vi "WaitAdjust.vi"(9 "PassthroughTime_SEC":dbl=-1.0, 10 "MaxAdjustment_MS":dbl=5.0, 11 "DesiredLoopTime_MS":dbl=20.0) -> (2 "AdjustedWaitTime_MS":u32, 3 "Offset_MS":dbl)   [LabVIEW 2019, in "Trajectory_Library.lvlib"]
doc: "This routine fine tunes the wait time for a loop to attempt to provide the loop with more consistent timing and lower jitter. \n\nInputs:\n -- Desired Loop time -- Int32 -- Desired loop time in milliseconds. (Optional. Default: 20.0)\n -- MaxAdjustment -- Int32 -- Maximum time in milliseconds to adjust the wait time. (Optional. Default: 5.0)\n -- PassthroughTime -- double float -- Elapsed time clock. (Optional. Default: Read FPGA clock)\n\nOutputs:\n -- Adjusted Wait Time -- Uint32 -- Updated wait time in milliseconds to feed to the wait VI.\n - Offset MS -- double float -- Current value of accumulated loop time error."
uses:
  Trajectory_Library.lvlib
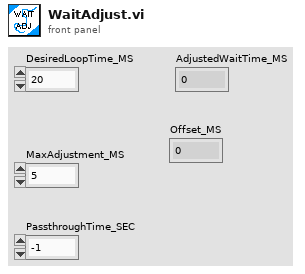
[diagram p1: front panel]
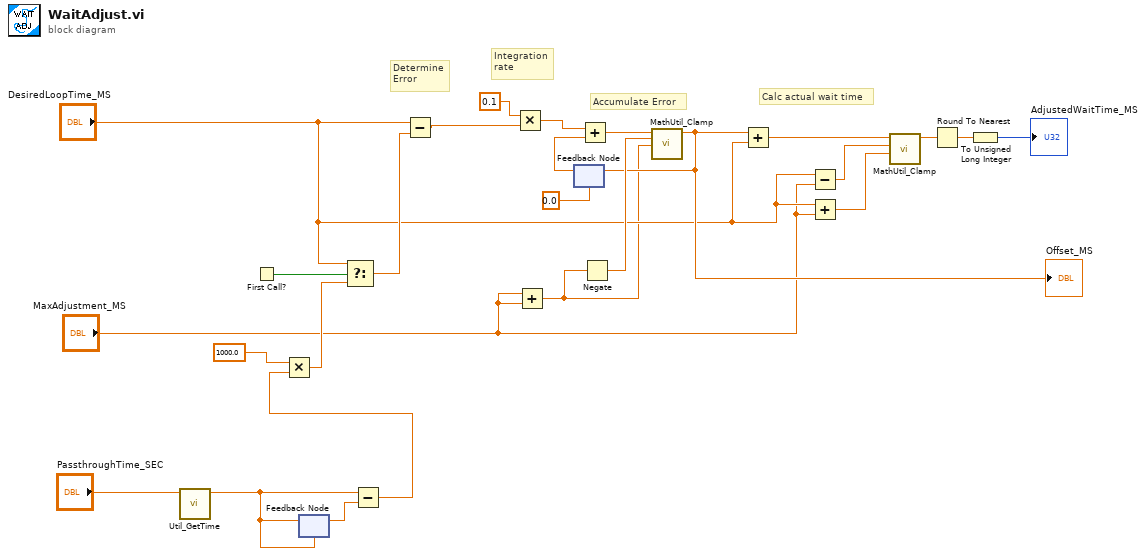
[diagram p0: block diagram]
diagram:
  # "Integration\nrate"
  # "Calc actual wait time"
  # "Determine\nError"
  # "Accumulate Error"
  n1 = call "Util_GetTime.vi"("Pass_Through_Time"="PassthroughTime_SEC") -> ("FPGA_Time_Seconds"=w7:dbl)  [unwired: 8 in, 2 out]
  n2 = First Call?() -> (First Call?: T/F=w12:bool)
  n3 = feedback-in #1(w7) -> ()
  n4 = feedback #1(w7) -> (w13:dbl)
  n5 = Subtract(x=w7, y=w13) -> (x-y=w6:dbl)
  n6 = Multiply(x=1000.0, y=w6) -> (x*y=w9:dbl)
  n7 = Select(t="DesiredLoopTime_MS", s=w12, f=w9) -> (s? t:f=w11:dbl)
  n8 = Subtract(x="DesiredLoopTime_MS", y=w11) -> (x-y=w2:dbl)
  n9 = Multiply(x=0.1, y=w2) -> (x*y=w3:dbl)
  n10 = Add(x="MaxAdjustment_MS", y="MaxAdjustment_MS") -> (x+y=w4:dbl)
  n11 = feedback #2(0.0) -> (w23:dbl)
  n12 = Add(x=w3, y=w23) -> (x+y=w24:dbl)
  n13 = Negate(x=w4) -> (-x=w18:dbl)
  n14 = call "MathUtil_Clamp.vi"("High Limit"=w4, "Low Limit"=w18, "Value"=w24) -> ("Result"=w15:dbl)  [unwired: 8 in]
  "Offset_MS" <- w15
  n15 = feedback-in #2(w15) -> ()
  n16 = Add(x=w15, y="DesiredLoopTime_MS") -> (x+y=w25:dbl)
  n17 = Subtract(x="DesiredLoopTime_MS", y="MaxAdjustment_MS") -> (x-y=w17:dbl)
  n18 = Add(x="DesiredLoopTime_MS", y="MaxAdjustment_MS") -> (x+y=w16:dbl)
  n19 = call "MathUtil_Clamp.vi"("High Limit"=w16, "Low Limit"=w17, "Value"=w25) -> ("Result"=w19:dbl)  [unwired: 8 in]
  n20 = Round To Nearest(number=w19) -> (nearest integer value=w20:dbl)
  n21 = To Unsigned Long Integer(number=w20) -> (unsigned 32bit integer=→"AdjustedWaitTime_MS":u32)
